vi "Configure_DO_Module.vi"(8 "error in (no error)":errorcluster, 10 "DO_Module_Data":T1 {"Module_Data"."Address" format="%x"}, 11 "USB-87Pn in":refnum<class "USB-87Pn.lvclass">) -> (0 "error out":errorcluster, 3 "USB-87Pn out":refnum<class "USB-87Pn.lvclass">)   [LabVIEW 2019, in "USB-87Pn.lvlib" / "USB-87Pn.lvclass"]
uses:
  USB-87Pn.lvclass
  Module/DO_Module_Data.ctl
  Module/Module_Data.ctl
  USB-87Pn.lvclass/USB-87Pn.ctl
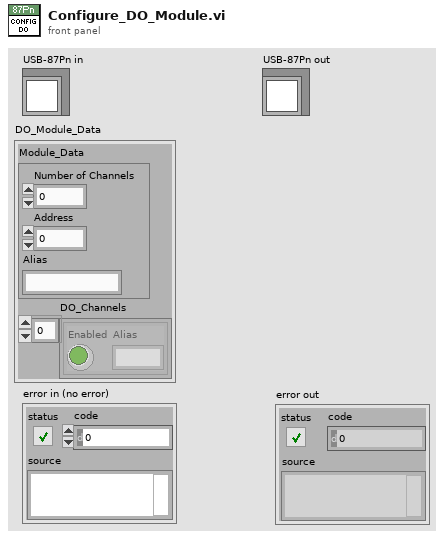
[diagram p1: front panel]
types:
  T1 = typedef "USB-87Pn.lvlib/USB-87Pn.lvclass/DO_Module_Data.ctl" = cluster{"Module_Data":T2, "DO_Channels":cluster{"Enabled":bool, "Alias":string}[]}
  T2 = typedef "USB-87Pn.lvlib/USB-87Pn.lvclass/Module_Data.ctl" = cluster{"Number of Channels":u8, "Address":i16, "Alias":string}
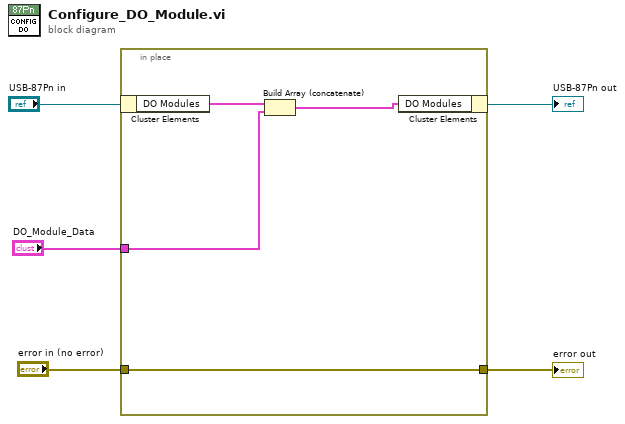
[diagram p0: block diagram]
diagram:
  n1 = in-place {
    in-place-border: "DO_Module_Data" -> [w8]
    in-place-border: "error in (no error)" -> [w7]
    in-place-border: [w7] -> w2
    n2 = in-place-cluster #1("USB-87Pn in") -> ("DO Modules"=w9:T1[])
    n3 = Build Array (concatenate)(w9, w8) -> (w6:T1[])
    n4 = in-place-cluster #1("DO Modules"=w6) -> (→"USB-87Pn out":refnum<class "USB-87Pn.lvclass">)
  }
  "error out" <- w2
